vi "Ini key read (String).vi"(7 "Section name":string, 8 "error in (no error)":errorcluster, 10 "Keys setup":T2, 11 "Ini file ref in":T1) -> (0 "error out":errorcluster, 2 "Value read/used":string[](array[string]), 3 "Ini file ref":T1)   [LabVIEW 2017]
uses:
  Typedefs/Ini file interface (String).ctl
  <vilib>/Utility/config.llb/Config Data RefNum.ctl
  <vilib>/Utility/config.llb/Read Key (String).vi
  <vilib>/Utility/config.llb/Write Key (String).vi
  <vilib>/Utility/config.llb/NI_LVConfig.lvlib
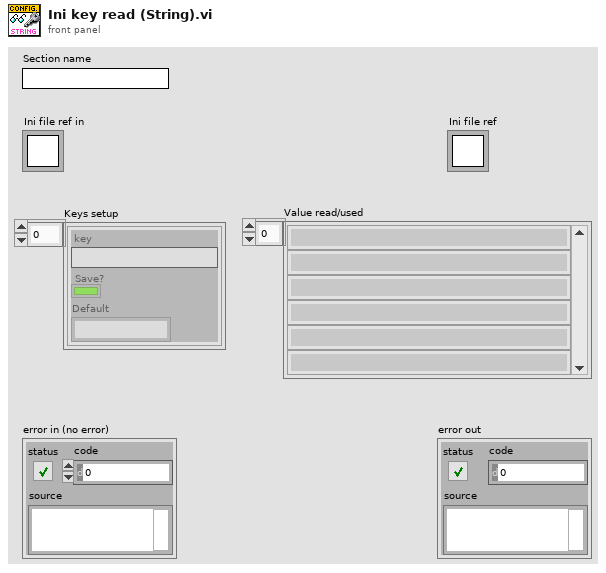
[diagram p1: front panel]
types:
  T1 = typedef "NI_LVConfig.lvlib/Config Data RefNum.ctl" = refnum<k1>
  T2 = typedef "Ini file interface (String).ctl" = cluster{"key":string, "Save?":bool, "Default":string}[]
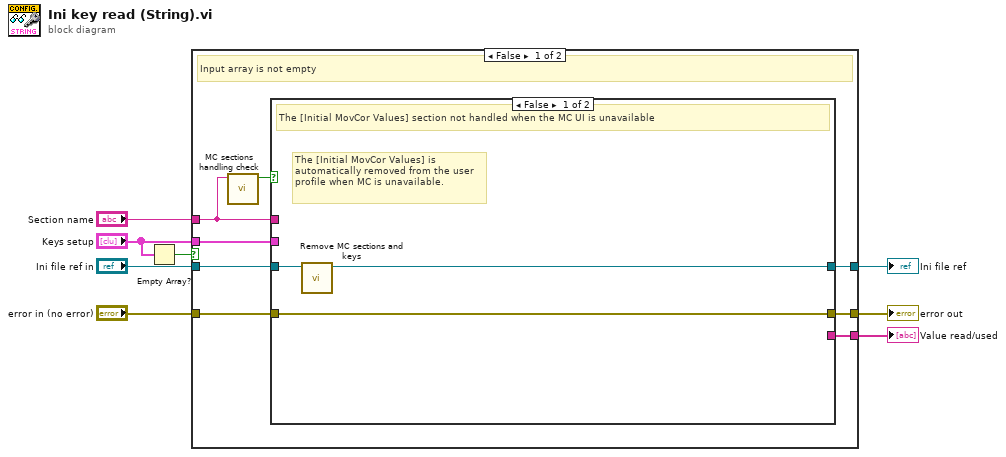
[diagram p0: block diagram]
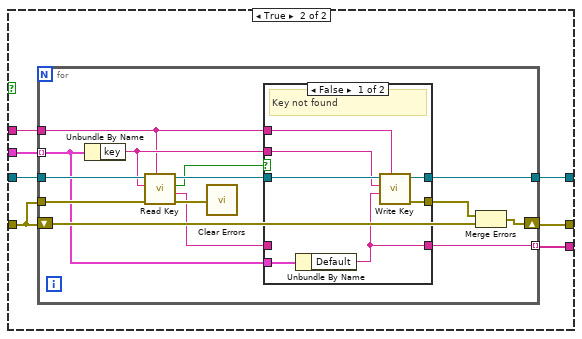
[diagram p2: hidden frame]
diagram:
  n1 = Empty Array?(array="Keys setup") -> (empty?=w1:bool)
  n2 = case shown="False" w1 {
    tunnel: "Section name" -> [w10 _]
    tunnel: "Keys setup" -> [w16 _]
    tunnel: [w15 _] -> w7
    tunnel: "error in (no error)" -> [w14 w50]
    tunnel: [w13 w50] -> w5
    tunnel: [w12 w51] -> w4
    tunnel: "Ini file ref in" -> [w11 w51]
    frame False {
      # "Input array is not empty"
      n3 = call "MC sections handling check.vi"("Section name"=w10) -> ("Section is \"Initial MovCor Values\" AND MC is supported"=w9:bool)  [unwired: 10 in]
      n4 = case shown="False" w9 {
        tunnel: w16 -> [_ w26]
        tunnel: [_ w25] -> w15
        tunnel: w14 -> [w19 w24]
        tunnel: [w19 w23] -> w13
        tunnel: [w17 w22] -> w12
        tunnel: w11 -> [w18 w21]
        tunnel: w10 -> [_ w20]
        frame False {
          # "The [Initial MovCor Values] is automatically removed from the user profile when MC is unavailable."
          # "The [Initial MovCor Values] section not handled when the MC UI is unavailable"
          n5 = call "Remove MC sections and keys.vi"("User profile ref"=w18) -> ("User profile ref"=w17:T1)  [unwired: 10 in]
        }
        frame True {
          n6 = for {
            tunnel: w20 -> [w27]
            tunnel: w21 -> [w40]
            tunnel: w24 -> [w39]
            tunnel: [w34] -> w22
            shift-right: [w38] -> w23
            shift-left: w24 -> [w37]
            tunnel: w26 -> [w28] mode=indexing
            tunnel: [w30] -> w25 mode=indexing
            n7 = Unbundle By Name(w28) -> ("key"=w29:string)
            n8 = call-poly <vilib>:"Read Key.vi"("section"=w27, "error in (no error)"=w39, "key"=w29, "refnum"=w40) -> ("error out"=w36:errorcluster, "value"=w31:string, "found?"=w32:bool, "refnum out"=w35:T1)  [unwired: 4 in]
            n9 = call <vilib>:"Clear Errors.vi"("error in (no error)"=w36) -> ()  [unwired: 5 in, 2 out]
            n10 = case shown="False" w32 {
              tunnel: w35 -> [w47 w49]
              tunnel: [w46 w49] -> w34
              tunnel: [w45 _] -> w33
              tunnel: w27 -> [w44 _]
              tunnel: w29 -> [w43 _]
              tunnel: w31 -> [_ w48]
              tunnel: [w41 w48] -> w30
              tunnel: w28 -> [w42 _]
              frame False {
                # "Key not found"
                n11 = Unbundle By Name(w42) -> ("Default"=w41:string)
                n12 = call-poly <vilib>:"Write Key.vi"("section"=w44, "value"=w41, "key"=w43, "refnum"=w47) -> ("error out"=w45:errorcluster, "refnum out"=w46:T1)  [unwired: 5 in, 1 out]
              }
              frame True {
                # "Key found"
              }
            }
            n13 = Merge Errors(w33, w37) -> (w38:errorcluster)
          }
        }
      }
    }
    frame True {
      # "Input array is empty"
    }
  }
  "Value read/used" <- w7
  "error out" <- w5
  "Ini file ref" <- w4
